vi "Sensor Reads.vi"   [LabVIEW 2020]
uses:
  <vilib>/Rock Robotics/WPI/ThirdParty/Phoenix-LabVIEW/CANCoder/Get/CTRE_Phoenix_CANcoder_GetSensorData.vi
types:
  T1 = typedef "WPI_MotorControlDeviceRef.ctl" = cluster{"DeviceStatus":errorcluster, "Type":T2, "PWM":cluster{"PWM Channel":T3, "DeadBand":T4}, "CAN":cluster{"Device Number":u8, "SetOutput VI Ref":variant, "GetOutput VI Ref":variant, "Enable VI Ref":variant, "Disable VI Ref":variant, "Data":variant}, "Invert":bool, "DIO PWM":cluster{"PWM \"Enable\" Channel":T3, "DIOChannel":T5, "PWM Rate":dbl}}
  T2 = typedef "WPI_MotorControlType.ctl" = enum16{"PWM", "CAN", "DIO PWM"}
  T3 = typedef "FPGA_DIOPWMChannel.ctl" = enum8{"PWM 0", "PWM 1", "PWM 2", "PWM 3", "PWM 4", "PWM 5", "PWM 6", "PWM 7", "PWM 8", "PWM 9", "PWM MXP 0", "PWM MXP 1", "PWM MXP 2", "PWM MXP 3", "PWM MXP 4", "PWM MXP 5", "PWM MXP 6", "PWM MXP 7", "PWM MXP 8", "PWM MXP 9", "Invalid"}
  T4 = typedef "WPI_PWMDeadband.ctl" = cluster{"Name":string, "maxPositivePwm":i32, "minPositivePwm":i32, "centerPwm":i32, "maxNegativePwm":i32, "minNegativePwm":i32, "angularRange":u16}
  T5 = typedef "FPGA_DIOChannel.ctl" = enum8{"DIO 0", "DIO 1", "DIO 2", "DIO 3", "DIO 4", "DIO 5", "DIO 6", "DIO 7", "DIO 8", "DIO 9", "DIO MXP 0", "DIO MXP 1", "DIO MXP 2", "DIO MXP 3", "DIO MXP 4", "DIO MXP 5", "DIO MXP 6", "DIO MXP 7", "DIO MXP 8", "DIO MXP 9", "DIO MXP 10", "DIO MXP 11", "DIO MXP 12", "DIO MXP 13", "DIO MXP 14", "DIO MXP 15", "SPI Port CS1", "SPI Port CS2", "SPI Port CS3", "SPI Port MISO", "SPI Port MOSI", "Invalid"}
  T6 = typedef "CTRE_Phoenix_CANcoder_DeviceRef.ctl" = cluster{"DeviceStatus":errorcluster, "Device Number":u8, "Handle":u64, "UsageFrame":u32, "Library Path":path}
  T7 = typedef "WPI_GyroDevRef.ctl" = cluster{"DevStatus":errorcluster, "Analog Channel":T8, "Gain (VoltsPerDegree/Second)":dbl, "Gyro Type":enum16{"Analog", "XRS450"}, "Handle":i32, "SPI Bus":T9, "Device Found":bool, "Sample Rate":dbl, "Calibrate On Open":bool, "Offset":dbl}
  T8 = typedef "FPGA_AIChannel.ctl" = enum8{"AI 0", "AI 1", "AI 2", "AI 3", "AI MXP 0", "AI MXP 1", "AI MXP 2", "AI MXP 3", "Invalid"}
  T9 = typedef "spi_bus.ctl" = enum16{"SPI On-Board, CS0", "SPI On-Board, CS1", "SPI On-Board, CS2", "SPI On-Board, CS3", "SPI MXP", "Invalid"}
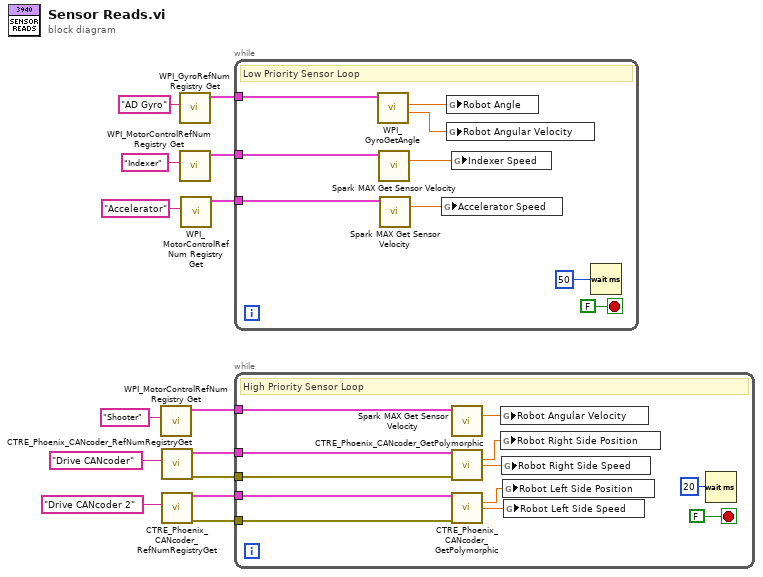
[diagram p0: block diagram]
diagram:
  n1 = call <vilib>:"WPI_MotorControlRefNum Registry Get.vi"("refnum name"="Shooter") -> ("MotorControlDevRef"=w1:T1)  [unwired: 9 in, 1 out]
  n2 = call <vilib>:"CTRE_Phoenix_CANcoder_RefNumRegistryGet.vi"("refnum name"="Drive CANcoder") -> ("error out"=w3:errorcluster, "CTRE_CANcoder_DeviceRef"=w2:T6)  [unwired: 9 in]
  n3 = call <vilib>:"CTRE_Phoenix_CANcoder_RefNumRegistryGet.vi"("refnum name"="Drive CANcoder 2") -> ("error out"=w5:errorcluster, "CTRE_CANcoder_DeviceRef"=w4:T6)  [unwired: 9 in]
  n4 = call <vilib>:"WPI_GyroRefNum Registry Get.vi"("refnum name"="AD Gyro") -> ("GyroDevRef"=w9:T7)  [unwired: 9 in, 1 out]
  n5 = call <vilib>:"WPI_MotorControlRefNum Registry Get.vi"("refnum name"="Indexer") -> ("MotorControlDevRef"=w10:T1)  [unwired: 9 in, 1 out]
  n6 = call <vilib>:"WPI_MotorControlRefNum Registry Get.vi"("refnum name"="Accelerator") -> ("MotorControlDevRef"=w11:T1)  [unwired: 9 in, 1 out]
  n7 = while {
    tunnel: w11 -> [w17]
    tunnel: w10 -> [w16]
    tunnel: w9 -> [w15]
    stop <- FALSE stop-if-true
    # "Low Priority Sensor Loop"
    n8 = call <vilib>:"WPI_GyroGetAngle.vi"("GyroDevRef"=w15) -> ("Angular Rate"=w20:dbl, "Angle"=w21:dbl)  [unwired: 6 in, 3 out]
    n9 = call <vilib>:"Spark MAX Get Sensor Velocity.vi"("MotorControlDevRef in"=w16) -> ("Sensor Velocity"=w19:dbl)  [unwired: 7 in, 3 out]
    n10 = call <vilib>:"Spark MAX Get Sensor Velocity.vi"("MotorControlDevRef in"=w17) -> ("Sensor Velocity"=w18:dbl)  [unwired: 7 in, 3 out]
    n11 = global write "Global Sensor Reads.vi" "Accelerator Speed"(w18) -> ()
    n12 = global write "Global Sensor Reads.vi" "Robot Angle"(w21) -> ()
    n13 = global write "Global Sensor Reads.vi" "Robot Angular Velocity"(w20) -> ()
    n14 = global write "Global Sensor Reads.vi" "Indexer Speed"(w19) -> ()
    n15 = Wait (ms)(milliseconds to wait=50) -> ()  [unwired: 1 out]
  }
  n16 = while {
    tunnel: w5 -> [w30]
    tunnel: w4 -> [w29]
    tunnel: w3 -> [w28]
    tunnel: w2 -> [w27]
    tunnel: w1 -> [w26]
    stop <- FALSE stop-if-true
    # "High Priority Sensor Loop"
    n17 = call <vilib>:"Spark MAX Get Sensor Velocity.vi"("MotorControlDevRef in"=w26) -> ("Sensor Velocity"=w35:dbl)  [unwired: 7 in, 3 out]
    n18 = call-poly <vilib>:"CTRE_Phoenix_CANcoder_GetPolymorphic.vi"("CTRE_CANcoder_DeviceRef"=w27, "error in"=w28) -> ("Position"=w25:dbl, "Velocity"=w34:dbl)  [unwired: 9 in, 3 out]
    n19 = call-poly <vilib>:"CTRE_Phoenix_CANcoder_GetPolymorphic.vi"("CTRE_CANcoder_DeviceRef"=w29, "error in"=w30) -> ("Position"=w24:dbl, "Velocity"=w33:dbl)  [unwired: 9 in, 3 out]
    n20 = global write "Global Sensor Reads.vi" "Robot Angular Velocity"(w35) -> ()
    n21 = global write "Global Sensor Reads.vi" "Robot Right Side Position"(w25) -> ()
    n22 = global write "Global Sensor Reads.vi" "Robot Right Side Speed"(w34) -> ()
    n23 = global write "Global Sensor Reads.vi" "Robot Left Side Position"(w24) -> ()
    n24 = global write "Global Sensor Reads.vi" "Robot Left Side Speed"(w33) -> ()
    n25 = Wait (ms)(milliseconds to wait=20) -> ()  [unwired: 1 out]
  }
